vi "SimulateMouseClick.vi"(7 "Move":bool, 8 "Error In":errorcluster, 10 "Y Position":i32, 11 "X Position":i32) -> ()   [LabVIEW 2014]
uses:
  User32.dll
panel:
  out "Error Out":errorcluster
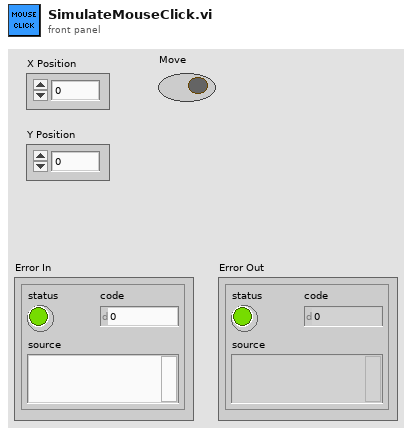
[diagram p1: front panel]
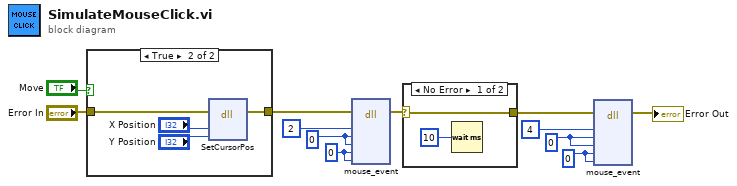
[diagram p0: block diagram]
diagram:
  w6 = 0 ("dwExtraInfo")
  w5 = u32 0 ("dwExtraInfo")
  w7 = 0 ("dwExtraInfo")
  w8 = u32 0 ("dwExtraInfo")
  n1 = case shown="True" "Move" {
    tunnel: [w13 w17] -> w10
    tunnel: "Error In" -> [w13 w14]
    frame False {
    }
    frame True {
      n2 = dll-call lib="user32.dll" fn="SetCursorPos" label="Move mouse"(error in=w14, "dx"="X Position", "dy"="Y Position") -> (error out=w17:errorcluster)  [unwired: 5 in, 1 out]
    }
  }
  n3 = dll-call lib="user32.dll" fn="mouse_event" label="Click"(error in=w10, "dwFlags"=2, "dx"=w7, "dy"=w7, "dwData"=w8, "dwExtraInfo"=w8) -> (error out=w11:errorcluster)  [unwired: 8 in, 1 out]
  n4 = case shown="No Error" w11 {
    selector: w11 -> [w18 w20]
    tunnel: [w18 w20] -> w12
    frame No Error {
      n5 = Wait (ms)(milliseconds to wait=u32 10) -> ()  [unwired: 1 out]
    }
    frame Error {
    }
  }
  n6 = dll-call lib="user32.dll" fn="mouse_event" label="Release"(error in=w12, "dwFlags"=4, "dx"=w6, "dy"=w6, "dwData"=w5, "dwExtraInfo"=w5) -> (error out=→"Error Out":errorcluster)  [unwired: 8 in, 1 out]
